vi "MotorBack 3(SubVI).vi"(11 "Cluster in 2":T1 {"Motor Step" items=["1 deg"=1, "3 deg"=3, "5 deg"=5, "10 deg"=10]; "Motor Range" items=["40 deg"=40, "360 deg"=360, "180 deg"=180]; "Mode" items=["Create", "Delete", "Select"]; "IF Bandwidth" format="%.3p"; "Span Freq" format="%.3p"; "Center Freq" format="%.3p"; "Power Level" format="%.2p"}) -> (3 "Cluster in 3":T1 {"Motor Step" items=["1 deg"=1, "3 deg"=3, "5 deg"=5, "10 deg"=10]; "Motor Range" items=["40 deg"=40, "360 deg"=360, "180 deg"=180]; "Mode" items=["Create", "Delete", "Select"]; "IF Bandwidth" format="%.3p"; "Span Freq" format="%.3p"; "Center Freq" format="%.3p"; "Power Level" format="%.2p"})   [LabVIEW 2020]
uses:
  Chamber_2018/ControlCluster.ctl
  D:/BWant RT/BWant_RT.lvlibp/Control Function.ctl
  D:/BWant RT/BWant_RT.lvlibp
panel:
  out "Locat 2":dbl caption="Current Location" format="%#.1f deg."
  in  "Stop 2":bool
  out "[ALM-A] 2":bool
  in  "Mode 2":enum16{"INC", "ABS"}(ring)=enum."ABS"
  out "[READY] 2":bool
  # "Hz"
  # "Hz"
  # "Hz"
  # "dBm"
  # "Hz"
  # "Hz"
  # "Hz"
  # "dBm"
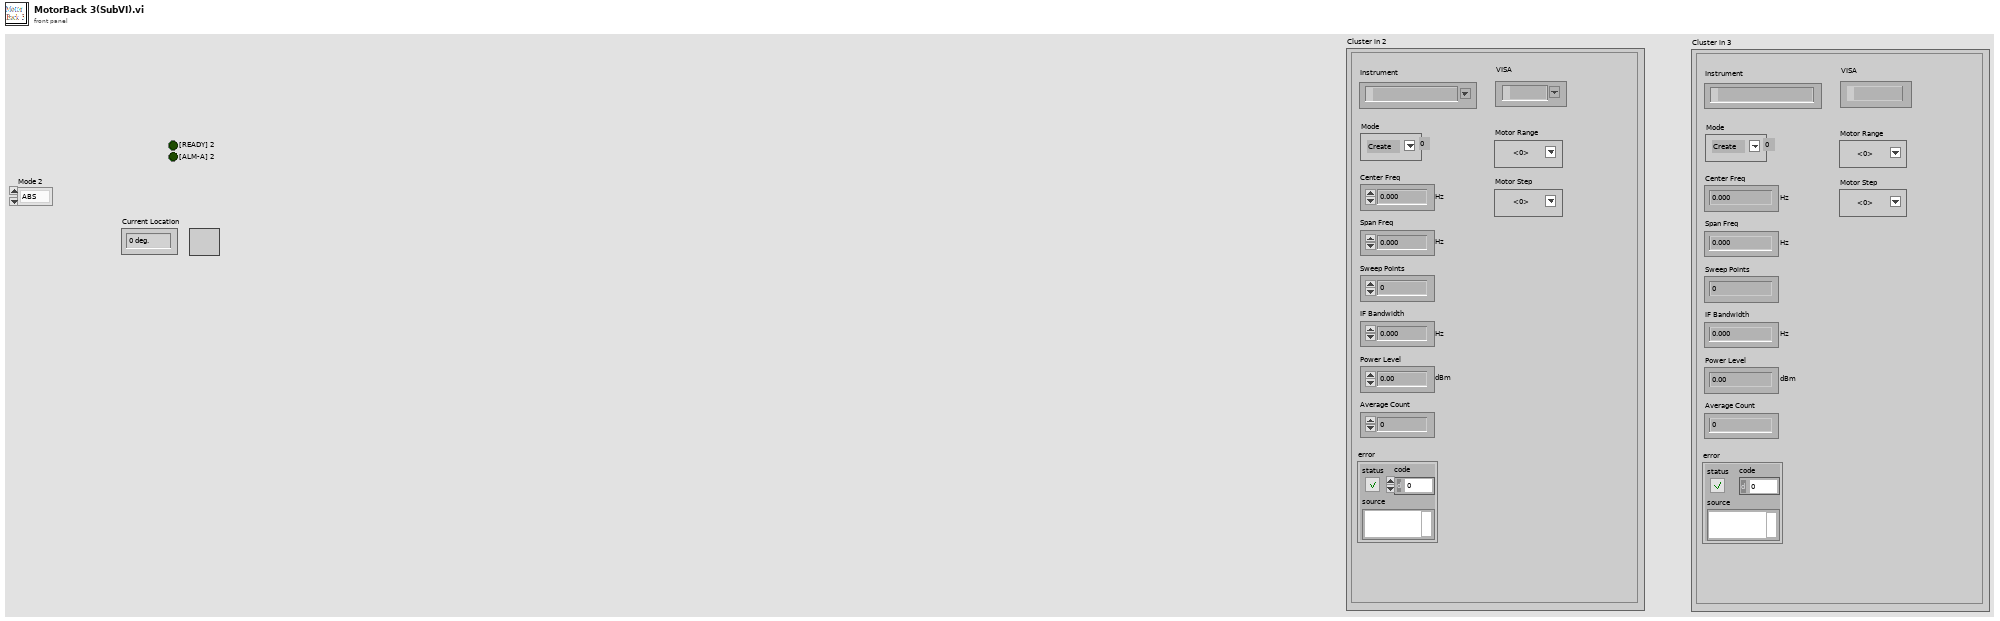
[diagram p1: front panel]
types:
  T1 = typedef "ControlCluster.ctl" = cluster{"Power Level":dbl, "Center Freq":dbl, "Span Freq":dbl, "Sweep Points":u32, "IF Bandwidth":dbl, "Average Count":i32, "error":errorcluster, "Instrument":refnum<visa-resource-name>, "Mode":u16, "Motor Range":u16, "Motor Step":u16, "VISA":refnum<visa-resource-name>}
  T2 = typedef "BWant_RT.lvlibp/Control Function.ctl" = enum16{"Idle", "Initial", "Close", "Check State", "ALM Reset", "ALM Inf", "Preset Home", "Pst_Value", "Speed", "Start-slope", "End-slpoe", "Read Pst", "GO Home", "Move", "Stop", "Limit mode", "MLU", "MLL", "Direction"}
  T3 = cluster{"[MOVE]":bool, "[READY]":bool, "[ALM-A]":bool}
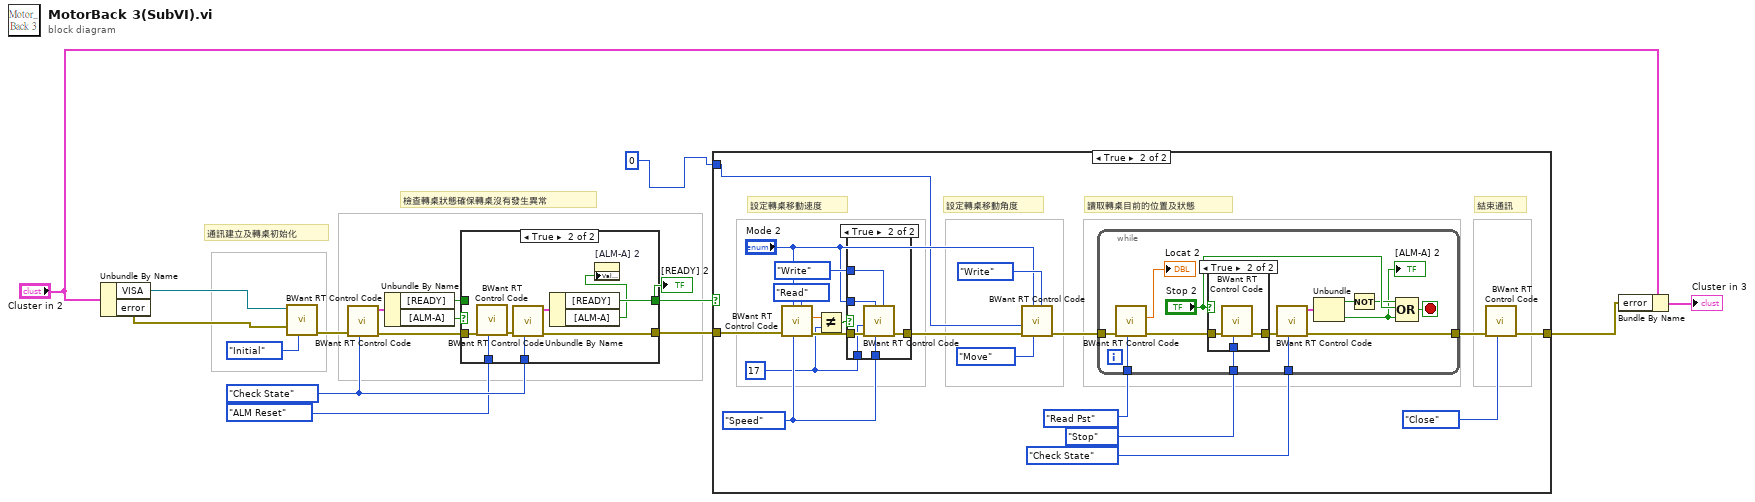
[diagram p0: block diagram]
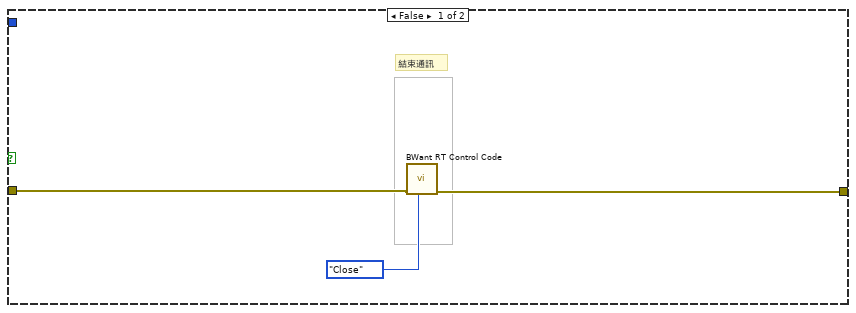
[diagram p2: hidden frame]
diagram:
  w8 = Control_Function."Check State" ("Fn")
  # "檢查轉桌狀態確保轉桌沒有發生異常"
  # "通訊建立及轉桌初始化"
  n1 = Unbundle By Name("Cluster in 2") -> ("VISA"=w6:refnum<visa-resource-name>, "error"=w5:errorcluster)
  n2 = call "BWant RT Control Code.vi"("Fn"=Control_Function."Initial", "error in"=w5, "ComPort"=w6) -> ("error out"=w13:errorcluster)  [unwired: 5 in, 3 out]
  n3 = call "BWant RT Control Code.vi"("Fn"=w8, "error in"=w13) -> ("error out"=w15:errorcluster, "State"=w14:T3)  [unwired: 6 in, 2 out]
  n4 = Unbundle By Name(w14) -> ("[READY]"=w12:bool, "[ALM-A]"=w16:bool)
  n5 = case shown="True" w16 {
    tunnel: [w18 w24] -> w11
    tunnel: w15 -> [w18 w20]
    tunnel: Control_Function."ALM Reset" ("Fn") -> [_ w26]
    tunnel: w8 -> [_ w23]
    tunnel: [w17 w21] -> w10
    tunnel: w12 -> [w17 _]
    frame False {
    }
    frame True {
      n6 = call "BWant RT Control Code.vi"("Fn"=w26, "error in"=w20) -> ("error out"=w25:errorcluster)  [unwired: 6 in, 3 out]
      n7 = call "BWant RT Control Code.vi"("Fn"=w23, "error in"=w25) -> ("error out"=w24:errorcluster, "State"=w22:T3)  [unwired: 6 in, 2 out]
      n8 = Unbundle By Name(w22) -> ("[READY]"=w21:bool, "[ALM-A]"=w19:bool)
      n9 = property on="[ALM-A] 2" class="Bool (strict)"("Value"=w19) -> ()  [unwired: 2 in, 2 out]
    }
  }
  "[READY] 2" <- w10
  n10 = case shown="True" w10 {
    tunnel: w11 -> [w29 w49]
    tunnel: [w28 w39] -> w2
    tunnel: 0 -> [_ w30]
    frame False {
      # "結束通訊"
      n11 = call "BWant RT Control Code.vi"("Fn"=Control_Function."Close", "error in"=w29) -> ("error out"=w28:errorcluster)  [unwired: 6 in, 3 out]
    }
    frame True {
      w31 = 17
      w37 = Control_Function."Speed" ("Fn")
      # "結束通訊"
      # "讀取轉桌目前的位置及狀態"
      # "設定轉桌移動角度"
      # "設定轉桌移動速度"
      n12 = call "BWant RT Control Code.vi"("Value_RW"=enum16{"Read", "Write"}."Read", "Fn"=w37, "Mode"="Mode 2", "error in"=w49) -> ("error out"=w47:errorcluster, "Value out"=w46:dbl)  [unwired: 4 in, 2 out]
      n13 = Not Equal?(x=w46, y=w31) -> (x != y?=w44:bool)
      n14 = case shown="True" w44 {
        tunnel: w47 -> [w68 w74]
        tunnel: w37 -> [_ w73]
        tunnel: w31 -> [_ w72]
        tunnel: enum16{"Read", "Write"}."Write" ("Value_RW") -> [_ w71]
        tunnel: [w68 w70] -> w42
        tunnel: "Mode 2" -> [_ w69]
        frame False {
        }
        frame True {
          n15 = call "BWant RT Control Code.vi"("Value_RW"=w71, "Fn"=w73, "Mode"=w69, "error in"=w74, "Value in"=w72) -> ("error out"=w70:errorcluster)  [unwired: 3 in, 3 out]
        }
      }
      n16 = call "BWant RT Control Code.vi"("Value_RW"=enum16{"Read", "Write"}."Write", "Fn"=Control_Function."Move", "Mode"="Mode 2", "error in"=w42, "Value in"=w30) -> ("error out"=w41:errorcluster)  [unwired: 3 in, 3 out]
      n17 = while {
        tunnel: w41 -> [w63]
        tunnel: Control_Function."Read Pst" ("Fn") -> [w62]
        tunnel: Control_Function."Stop" ("Fn") -> [w59]
        tunnel: Control_Function."Check State" ("Fn") -> [w57]
        tunnel: [w55] -> w40
        stop <- w51 stop-if-true
        n18 = call "BWant RT Control Code.vi"("Fn"=w62, "error in"=w63) -> ("error out"=w60:errorcluster, "Value out"=→"Locat 2":dbl)  [unwired: 6 in, 2 out]
        n19 = case shown="True" "Stop 2" {
          tunnel: w60 -> [w64 w67]
          tunnel: w59 -> [_ w66]
          tunnel: [w64 w65] -> w58
          frame False {
          }
          frame True {
            n20 = call "BWant RT Control Code.vi"("Fn"=w66, "error in"=w67) -> ("error out"=w65:errorcluster)  [unwired: 6 in, 3 out]
          }
        }
        n21 = call "BWant RT Control Code.vi"("Fn"=w57, "error in"=w58) -> ("error out"=w55:errorcluster, "State"=w56:T3)  [unwired: 6 in, 2 out]
        n22 = Unbundle(w56) -> ("[MOVE]"=w54:bool, "[ALM-A]"=w50:bool)  [unwired: 1 out]
        "[ALM-A] 2" <- w50
        n23 = Not(x=w54) -> (.not. x?=w52:bool)
        n24 = Compound Arithmetic op=OR(w52, "Stop 2", w50) -> (w51:bool)
      }
      n25 = call "BWant RT Control Code.vi"("Fn"=Control_Function."Close", "error in"=w40) -> ("error out"=w39:errorcluster)  [unwired: 6 in, 3 out]
    }
  }
  n26 = Bundle By Name(cluster="Cluster in 2", "error"=w2) -> (→"Cluster in 3":T1)
